vi "Delete empty string in a array.vi"(7 "Array in":string[](array[string])) -> (8 "Array out":string[](array[string]))   [LabVIEW 2012]
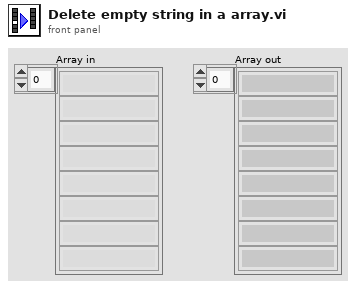
[diagram p1: front panel]
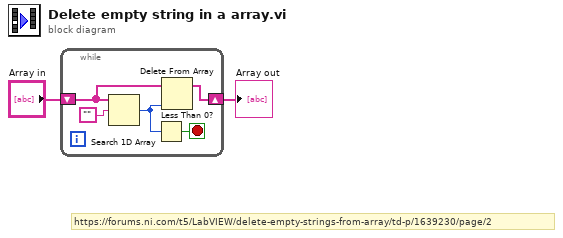
[diagram p0: block diagram]
diagram:
  # "https://forums.ni.com/t5/LabVIEW/delete-empty-strings-from-array/td-p/1639230/page/2"
  n1 = while {
    shift-right: [w4] -> w1
    shift-left: "Array in" -> [w6]
    stop <- w7 stop-if-true
    n2 = Search 1D Array(1D array=w6, element="") -> (index of element=w5:i32)  [unwired: 1 in]
    n3 = Less Than 0?(x=w5) -> (x < 0?=w7:bool)
    n4 = Delete From Array(array=w6, index=w5) -> (array with subset deleted=w4:string[])  [unwired: 1 in, 1 out]
  }
  "Array out" <- w1
